vi "CM-Read Hide Unused.vi"(0 "configuration file path":path=path "C:/PXI Connections.txt", 11 "error in (no error)":errorcluster) -> (4 "file path":path, 10 "Hide unused":bool, 15 "error out":errorcluster)   [LabVIEW 2020]
uses:
  Utility VIs/File IO VIs/Configuration File Wrapper VIs/Config-Read Key (Boolean).vi
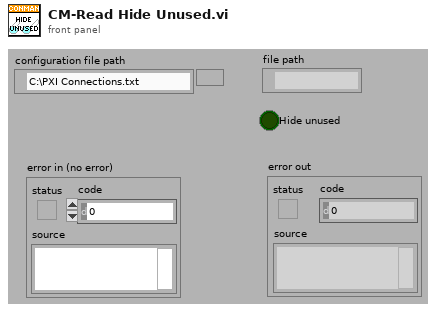
[diagram p1: front panel]
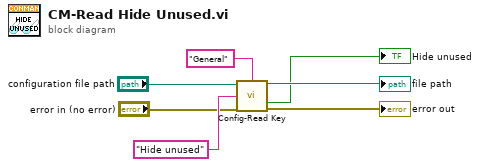
[diagram p0: block diagram]
diagram:
  n1 = call-poly "Config-Read Key.vi"("configuration file path"="configuration file path", "section"="General", "key"="Hide unused", "error in (no error)"="error in (no error)") -> ("file path"=→"file path":path, "value"=→"Hide unused":bool, "error out"=→"error out":errorcluster)  [unwired: 8 in, 1 out]
